vi "Newton_Stop Criteria.vi"(9 "dx":dbl, 10 "x0":dbl, 11 "noise":i32) -> (3 "stop if true":bool)   [LabVIEW 2020, in "NI_AALPro.lvlib"]
uses:
  NI_AALPro.lvlib
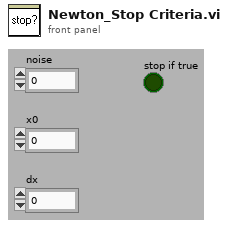
[diagram p1: front panel]
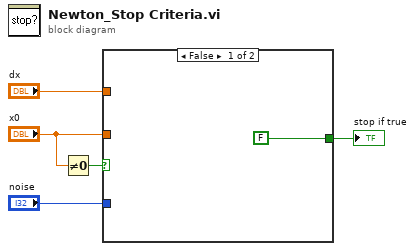
[diagram p0: block diagram]
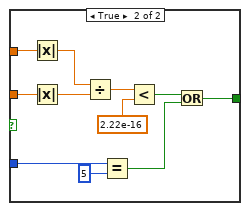
[diagram p2: hidden frame]
diagram:
  n1 = Not Equal To 0?(x="x0") -> (x != 0?=w5:bool)
  n2 = case shown="False" w5 {
    tunnel: "x0" -> [_ w17]
    tunnel: "dx" -> [_ w16]
    tunnel: "noise" -> [_ w12]
    tunnel: [FALSE w7] -> w1
    frame False {
    }
    frame True {
      n3 = Absolute Value(x=w16) -> (abs(x)=w9:dbl)
      n4 = Absolute Value(x=w17) -> (abs(x)=w15:dbl)
      n5 = Divide(x=w9, y=w15) -> (x/y=w8:dbl)
      n6 = Equal?(x=w12, y=5) -> (x = y?=w10:bool)
      n7 = Less?(x=w8, y=2.22e-16 ("2^x")) -> (x < y?=w13:bool)
      n8 = Or(x=w13, y=w10) -> (x .or. y?=w7:bool)
    }
  }
  "stop if true" <- w1
